vi "HAL_Set Reference.vi"(8 "error in":errorcluster, 10 "External?":bool=TRUE, 11 "Handle In":T1) -> (0 "error out":errorcluster, 3 "Handle Out":T1)   [LabVIEW 2015]
uses:
  Handle.ctl
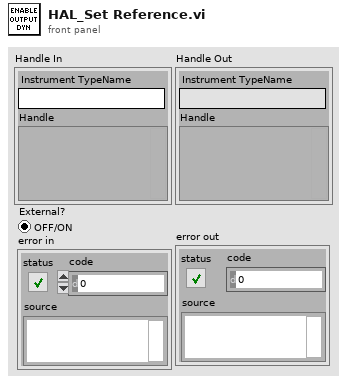
[diagram p1: front panel]
types:
  T1 = typedef "Handle.ctl" = cluster{"Instrument TypeName":string, "Handle":variant}
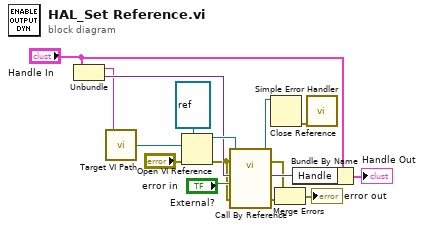
[diagram p0: block diagram]
diagram:
  n1 = Unbundle("Handle In") -> ("Instrument TypeName"=w5:string, "Handle"=w13:variant)
  n2 = call "Target VI Path.vi"("Instrument Name"=w5) -> ("Path to VI"=w6:path)
  n3 = Open VI Reference(type specifier VI Refnum (for type only)=refnum<vi> refnum, vi path=w6, error in (no error)="error in") -> (vi reference=w15:refnum<vi>, error out=w3:errorcluster)  [unwired: 3 in]
  n4 = call-by-ref "?"(reference=w15, error in=w3, "error in"=w3, "Enable?"="External?", "Handle In"=w13) -> (reference out=w1:refnum<vi>, error out=w9:errorcluster, 0:"error out"=w8:errorcluster, "Handle Out"=w11:variant)  [unwired: 7 in]
  n5 = Close Reference(reference=w1) -> (error out=w2:errorcluster)  [unwired: 1 in]
  n6 = Merge Errors(w9, w8) -> (→"error out":errorcluster)
  n7 = Bundle By Name(cluster="Handle In", "Handle"=w11) -> (→"Handle Out":T1)
  n8 = call <vilib>:"Simple Error Handler.vi"("error in (no error)"=w2) -> ()  [unwired: 4 in, 5 out]
